vi "requestFixedData.vi"(8 "error in (no error)":errorcluster, 9 "File name wo extension":string="AdminConfig", 10 "Fixed data type":T1=10 items=["Controller Configuration"=5, "Laser Configuration"=6, "Lens Configuration"=2, "Correction Table"=13, "User Configuration"=15, "Performance Adjustments"=16, "Admin Configuration"=10], 11 "SM1000-control in":T2) -> (0 "error out":errorcluster, 2 "File contents":string, 3 "SM1000-control out":T2)   [LabVIEW 2013, in "SLMControl.lvlib" / "SM1000.lvclass"]
doc: "Retrieve fixed data from an EC device session.\n\nEC1000 modules are autonomous devices that contain information that configures the module at boot-up for the particular hardware arrangement of the marking head. This information defines such things as the laser interface, the lens characteristics, and the optical system correction tables. An application can access this information by specifying the data type using the 'DataType' argument and providing a file name for the data as stored on the EC1000. The information is returned as an XML string which must be decoded by the application."
uses:
  SM1000.lvclass
  Object-reference.ctl
  Fixed-data-type.ctl
  SM1000.lvclass/SM1000.ctl
  Custom-errors.ctl
  C:/Users/vangeste/Desktop/2015-06-02 - SLM - MAIF/HC-HardwareCharacterization/Sources/SM1000/LECSession.dll
  HC-HardwareCharacterization/Sources/SM1000/LECSession.dll
  DOTNET-error-int.vi
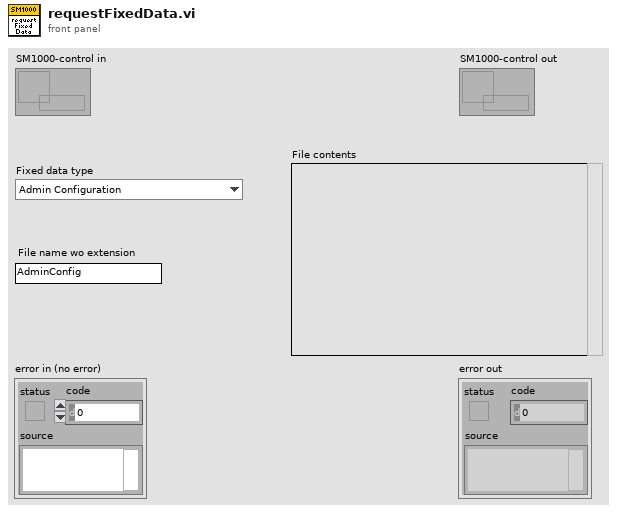
[diagram p1: front panel]
types:
  T1 = typedef "SLMControl.lvlib/SM1000.lvclass/Fixed-data-type.ctl" = i32
  T2 = typedef "SLMControl.lvlib/SM1000.lvclass/Object-reference.ctl" = refnum<data-value>
  T3 = typedef "SLMControl.lvlib/SM1000.lvclass/Custom-errors.ctl" = enum16{"No error", "Not implemented", "Command not recognized", "Invalid input", "No connection", "Timeout", "Resource not loaded"}
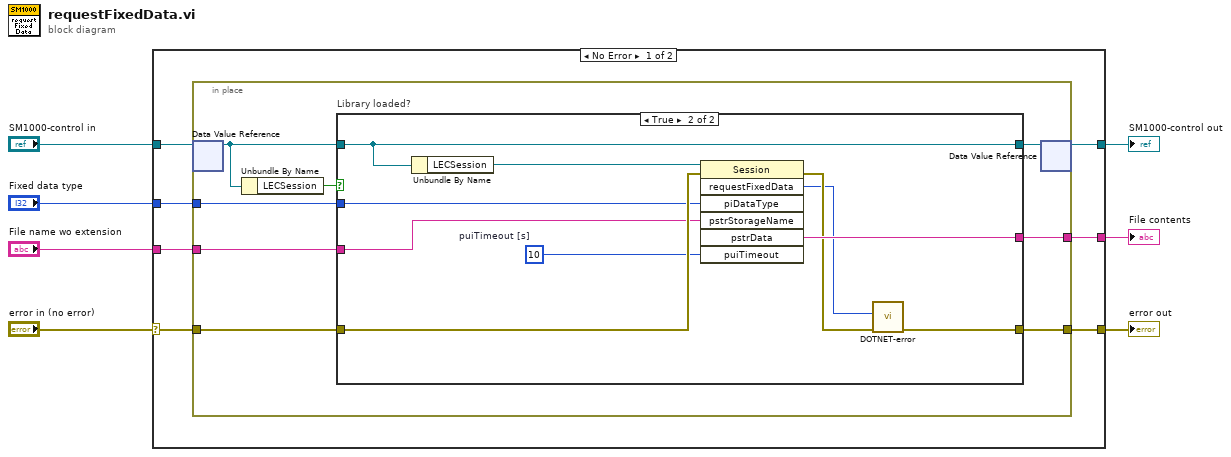
[diagram p0: block diagram]
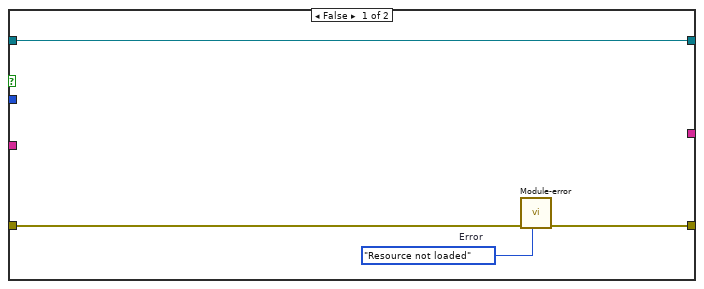
[diagram p2: hidden frame]
diagram:
  n1 = case shown="No Error" "error in (no error)" {
    selector: "error in (no error)" -> [w12 w38]
    tunnel: [w11 w38] -> w6
    tunnel: [w13 w37] -> w4
    tunnel: "SM1000-control in" -> [w14 w37]
    tunnel: "Fixed data type" -> [w10 _]
    tunnel: "File name wo extension" -> [w9 _]
    tunnel: [w8 _] -> w1
    frame No Error {
      n2 = in-place {
        in-place-border: w12 -> [w22]
        in-place-border: [w19] -> w11
        in-place-border: w10 -> [w17]
        in-place-border: w9 -> [w16]
        in-place-border: [w15] -> w8
        n3 = in-place-dvr #1(w14) -> (w20:refnum<class "SM1000.lvclass">)  [unwired: 1 out]
        n4 = Unbundle By Name(w20) -> ("LECSession"=w21:bool)
        n5 = case "Library loaded?" shown="True" w21 {
          tunnel: w22 -> [w26 w35]
          tunnel: w20 -> [w24 w31]
          tunnel: [w25 w29] -> w19
          tunnel: [w24 w31] -> w18
          tunnel: w17 -> [_ w33]
          tunnel: w16 -> [_ w32]
          tunnel: [_ w30] -> w15
          frame False {
            w23 = Custom-errors."Resource not loaded"  # Error
            n6 = call "Module-error.vi"("Error"=w23, "error in (no error)"=w26) -> ("error out"=w25:errorcluster)  [unwired: 9 in]
          }
          frame True {
            w34 = u32 10  # puiTimeout [s]
            n7 = Unbundle By Name(w31) -> ("LECSession"=w36:refnum<k24>)
            n8 = invoke class="Session" method="requestFixedData"(reference=w36, error in=w35, "piDataType"=w33, "pstrStorageName"=w32, "puiTimeout"=w34) -> (error out=w28:errorcluster, "requestFixedData"=w27:u32, "pstrData"=w30:string)  [unwired: 2 in, 4 out]
            n9 = call-poly "DOTNET-error.vi"("error in (no error)"=w28, "Retun code"=w27) -> ("error out"=w29:errorcluster)  [unwired: 9 in]
          }
        }
        n10 = in-place-dvr #1(w18) -> (w13:T2)  [unwired: 1 out]
      }
    }
    frame Error {
    }
  }
  "error out" <- w6
  "SM1000-control out" <- w4
  "File contents" <- w1
